vi "CR-导丝纤维毛发检测1.vi"(8 "error in (no error)":errorcluster caption="错误输入（无错误）", 11 "名称或相对路径":string="Template Program") -> (0 "error in (no error) 2":errorcluster caption="错误输入（无错误）")   [LabVIEW 2017]
uses:
  Picture/SaveButtom.ctl
  <vilib>/userdefined/High Color/IMAQdx.ctl
  <vilib>/vision/Pattern Matching.llb/IMAQ Curve Parameters.ctl
  Global System.vi
  <vilib>/Utility/xml.llb/Write to XML File(string).vi
panel:
  in  "相机选择":T1="cam0" caption="Session Out CCD3"
  in  "获取图像":bool
  in  "创建模板":bool
  in  "保存图像":bool
  out "添加的路径":path
  in  "刷新":bool
  in  "测试按钮":bool
  in  "保存按钮":bool
  in  "Main":enum32{"主参数", "颜色模板匹配参数 ", "测试效果"}(tab)
  in  "纤维毛发检测1基础参数":T2={"IsNorImage"=TRUE, "Exposure Values"=100289, "ImagePath"=path "C:/Users/hedongpo/Desktop/514-hdp/Alignment Assemble System/Test Picture/B/3.bmp", "相机选择"="cam0"} caption="参数界面" {"Exposure Values" scale=0.0..200000.0}
  in  "纤维毛发检测1参数":T4={"Curve Extraction Settings "={"Extraction Mode"=0, "Edge Threshold"=25, "Edge Filter Size"=1, "Min Length"=19, "Row Search Step Size"=5, "Col Search Step Size"=5, "Max Endpoint Gap"=10, "Closed"=FALSE, "Subpixel"=FALSE}, "Color Mode (Histogram 1)"=0, "Range (Threshold 1)"={"Lower value"=62.0, "Upper value"=255.0}, "Clamp Settings (Max Clamp 1)"={"Angle Range (+/-)"=10.0, "Edge Polarity"={"Start"=0, "End"=0}}, "Settings (Clamp (Rake) 1)"={"Contrast"=14, "Filter width"=14, "Steepness"=1, "Subsampling Ratio"=5, "Show Search Area"=FALSE, "Show Search Lines"=FALSE, "Show Edges Found"=TRUE, "Show Result"=TRUE}, "直径设定"={"Lower value"=62.0, "Upper value"=255.0}} {"Clamp Settings (Max Clamp 1)"."Edge Polarity"."Start" items=["Any", "Rising", "Falling"]; "Clamp Settings (Max Clamp 1)"."Edge Polarity"."End" items=["Any", "Rising", "Falling"]; "Color Mode (Histogram 1)" items=["RGB", "HSL", "HSV", "HSI"]; "Curve Extraction Settings"."Extraction Mode" items=["Normal", "Uniform Regions"]; "Curve Extraction Settings"."Edge Filter Size" items=["Fine", "Normal", "Contour Tracing"]; "Curve Extraction Settings"."Max Endpoint Gap" min=0; "Curve Extraction Settings"."Col Search Step Size" min=1 max=255 step=1; "Curve Extraction Settings"."Row Search Step Size" min=1 max=255 step=1; "Curve Extraction Settings"."Min Length" min=0; "Curve Extraction Settings"."Edge Threshold" min=1 max=350 step=1}
  out "结果":bool
  out "原始图像":T5(plugin-control)
  out "Distance (Clamp (Rake) 1)":sgl format="%.2f"
  out "路径输出":path
  in  "Vision Paramter Save Buttom":T6
  out "system time":string
  in  "取消按钮":bool
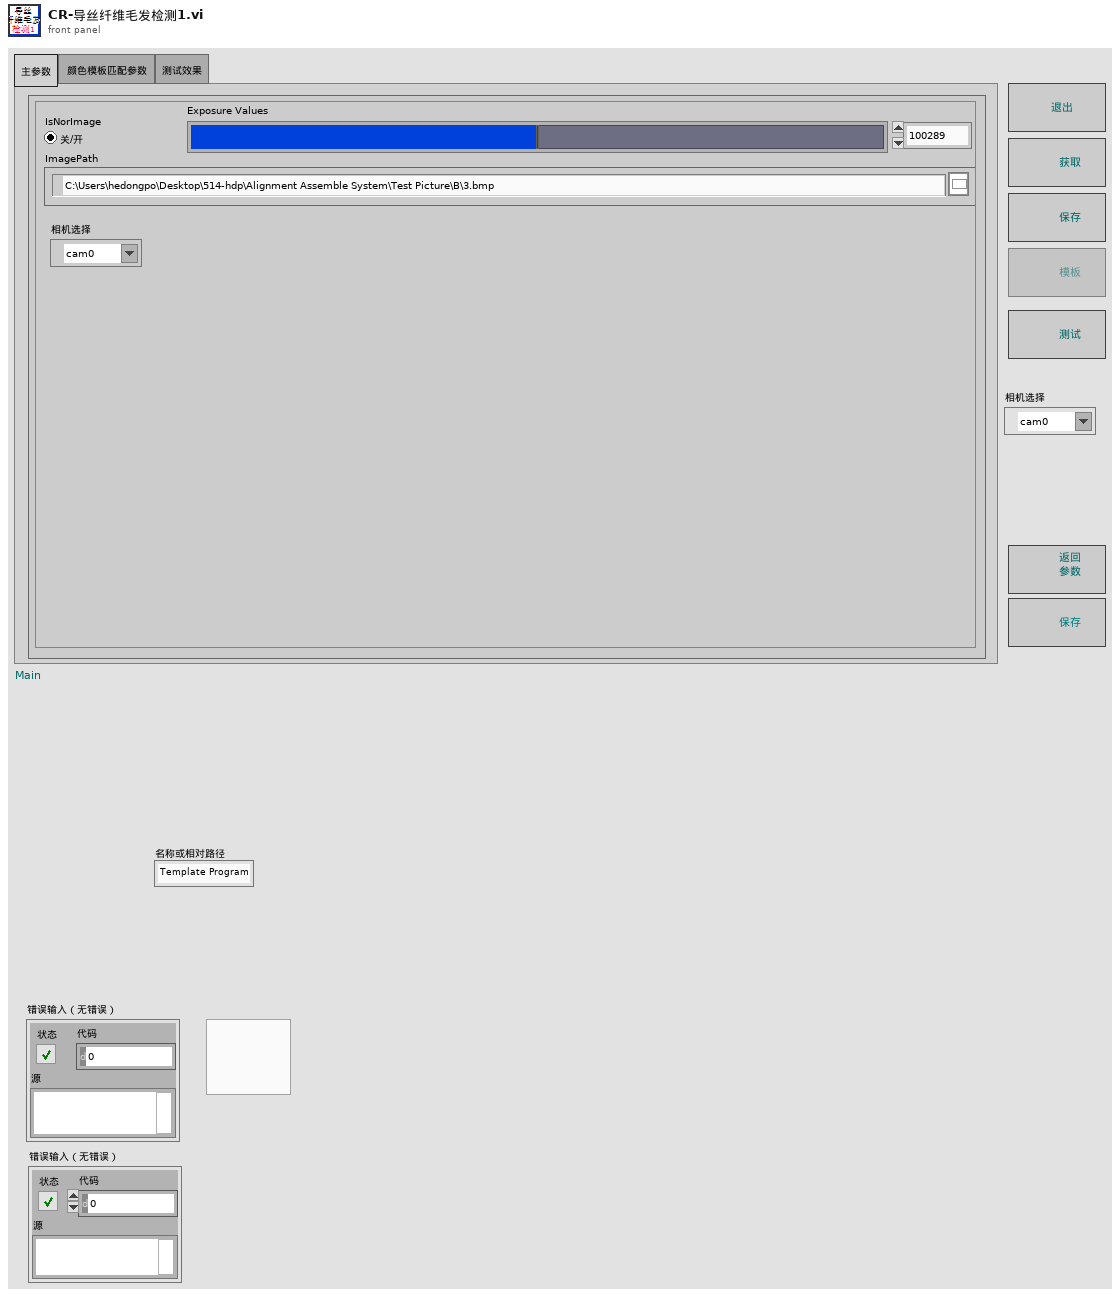
[diagram p1: front panel]
types:
  T1 = typedef "IMAQdx.ctl" = refnum<k21>
  T2 = cluster{"IsNorImage":bool, "Exposure Values":u32, "ImagePath":path, "相机选择":T1}
  T3 = typedef "IMAQ Curve Parameters.ctl" = cluster{"Extraction Mode":u32, "Edge Threshold":i32, "Edge Filter Size":u32, "Min Length":i32, "Row Search Step Size":i32, "Col Search Step Size":i32, "Max Endpoint Gap":i32, "Closed":bool, "Subpixel":bool}
  T4 = cluster{"Curve Extraction Settings ":T3, "Color Mode (Histogram 1)":u16, "Range (Threshold 1)":cluster{"Lower value":sgl, "Upper value":sgl}, "Clamp Settings (Max Clamp 1)":cluster{"Angle Range (+/-)":dbl, "Edge Polarity":cluster{"Start":u32, "End":u32}}, "Settings (Clamp (Rake) 1)":cluster{"Contrast":i32, "Filter width":i32, "Steepness":i32, "Subsampling Ratio":u32, "Show Search Area":bool, "Show Search Lines":bool, "Show Edges Found":bool, "Show Result":bool}, "直径设定":cluster{"Lower value":sgl, "Upper value":sgl}}
  T5 = typedef "IMAQ Image.ctl" = refnum<image>
  T6 = typedef "SaveButtom.ctl" = bool
  T7 = cluster{"index":i32, "this vi":refnum<vi>, "error out":errorcluster}
  T8 = cluster{"master data":string, "priority":u16, "secondary data":string[]}
  T9 = cluster{"case name":string[], "queue array":refnum<queue>[]}
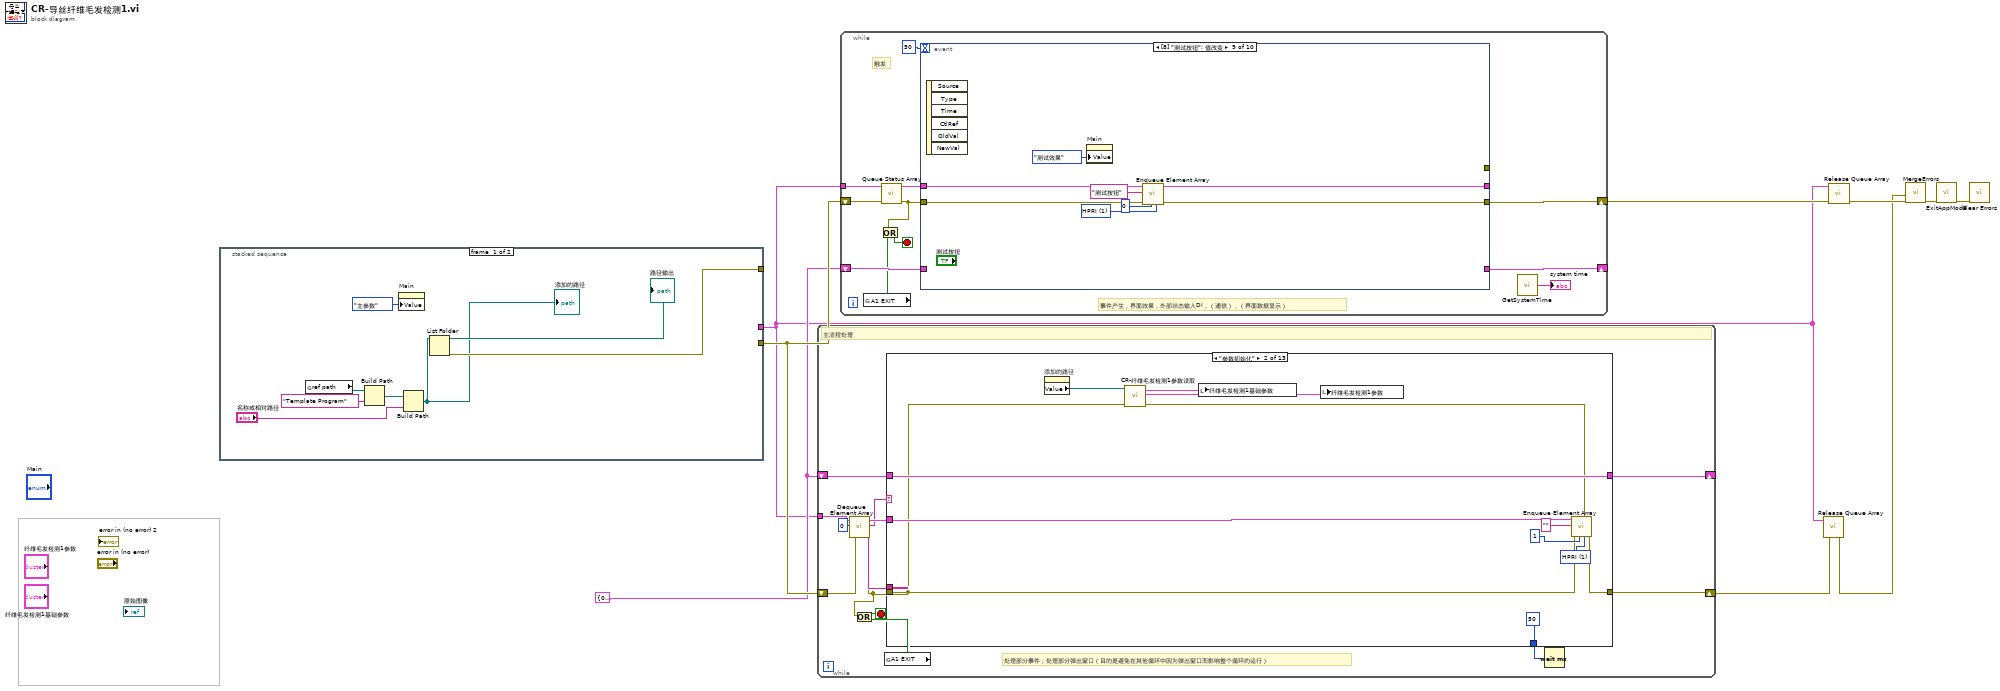
[diagram p0: block diagram]
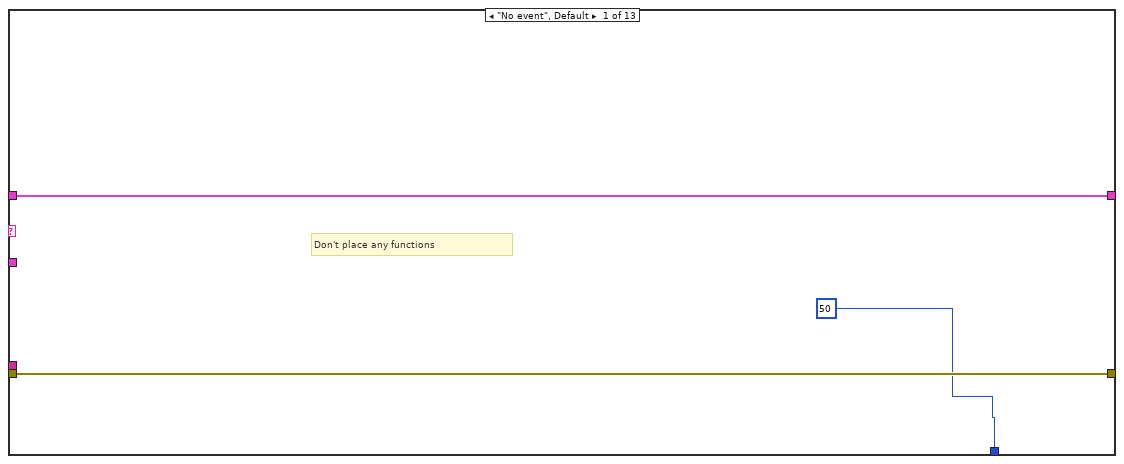
[diagram p2: hidden frame]
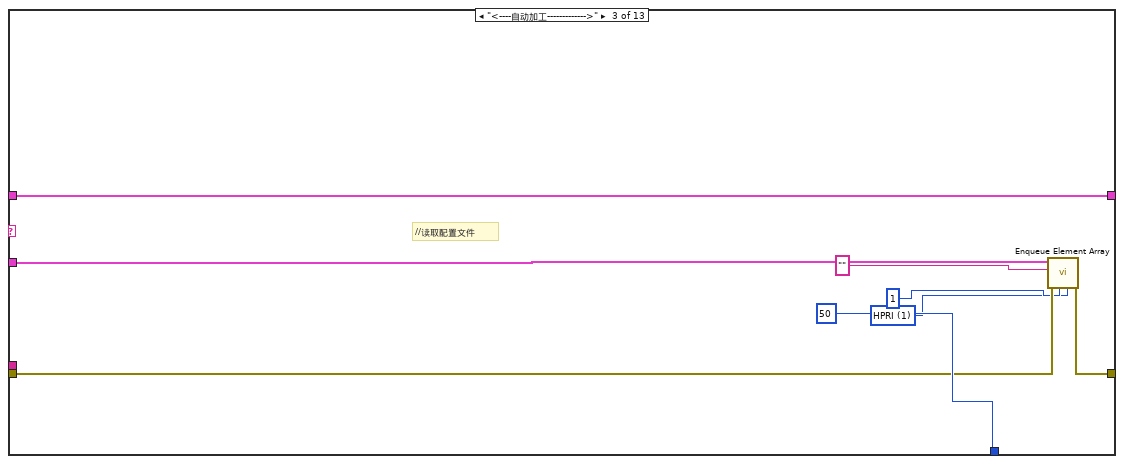
[diagram p3: hidden frame]
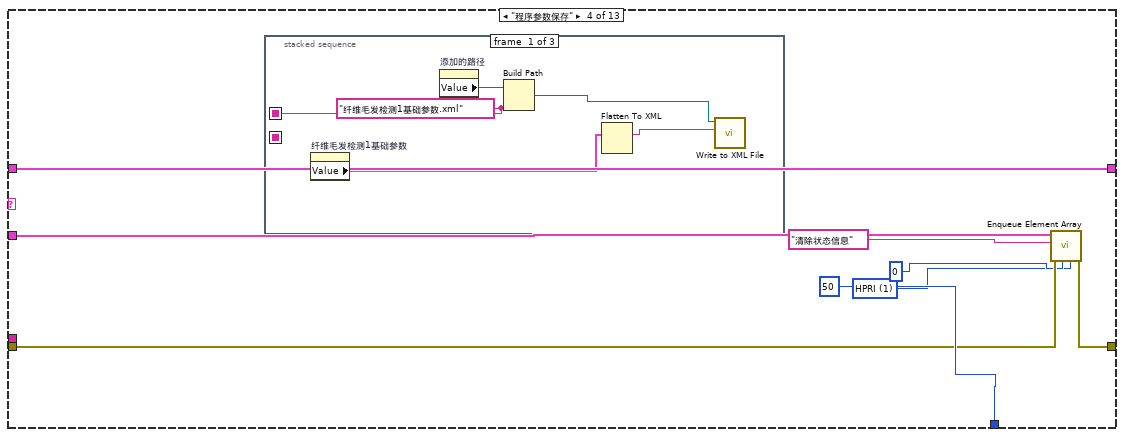
[diagram p4: hidden frame]
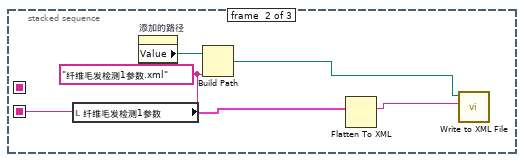
[diagram p5: hidden frame]
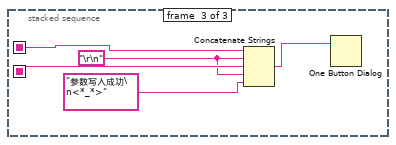
[diagram p6: hidden frame]
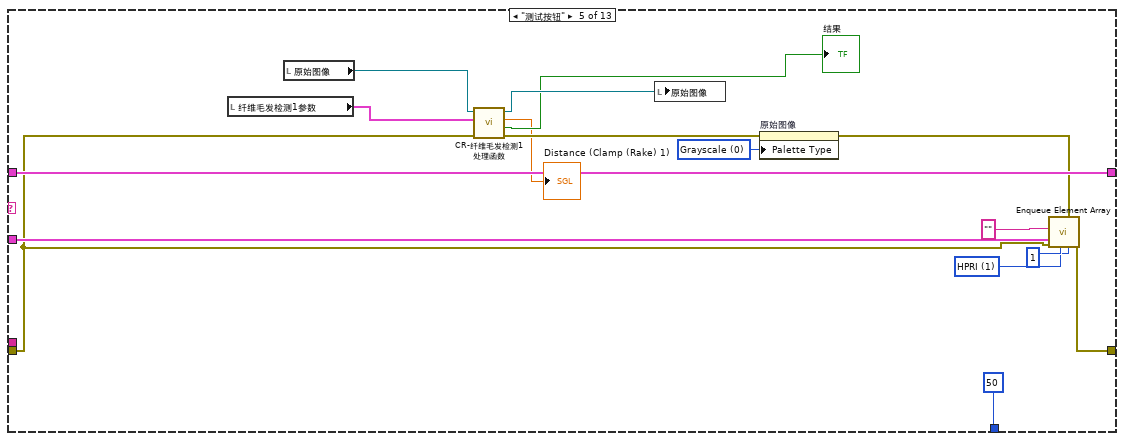
[diagram p7: hidden frame]
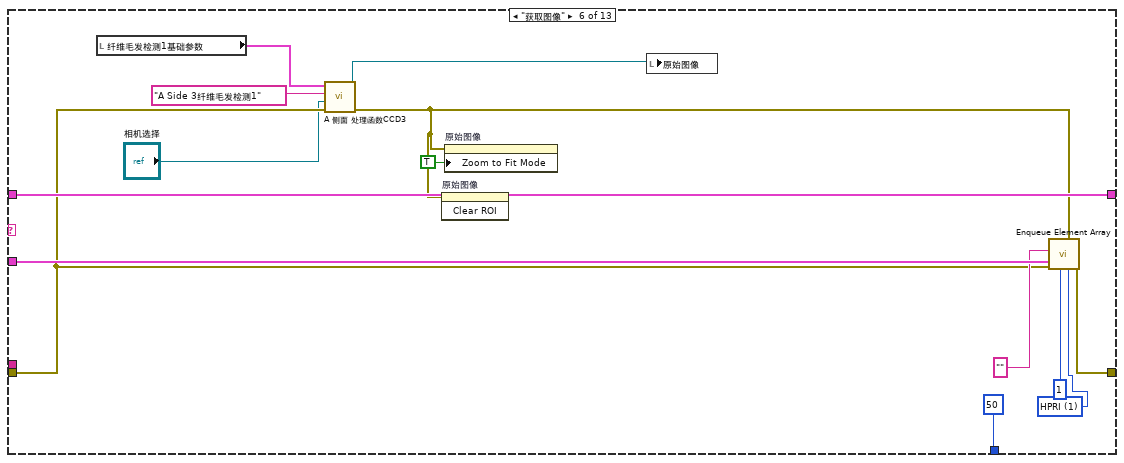
[diagram p8: hidden frame]
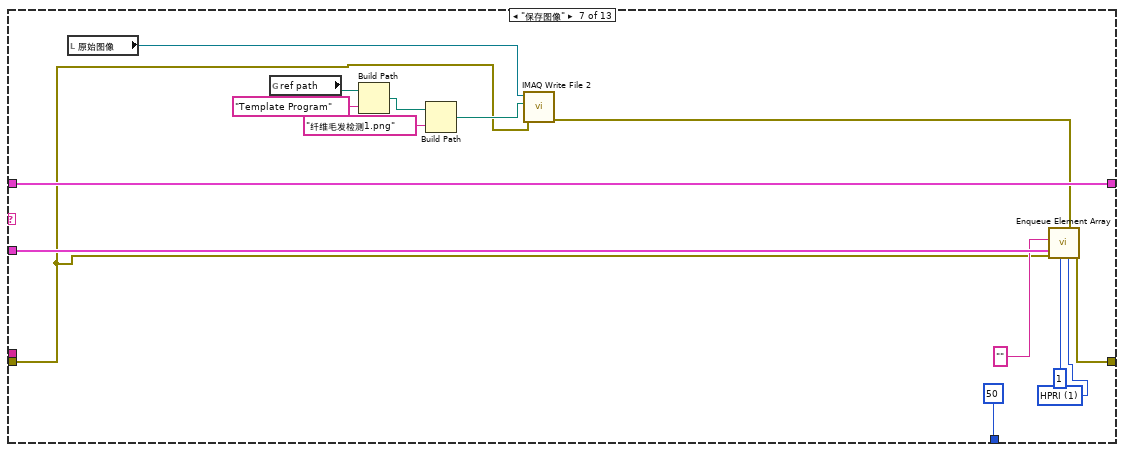
[diagram p9: hidden frame]
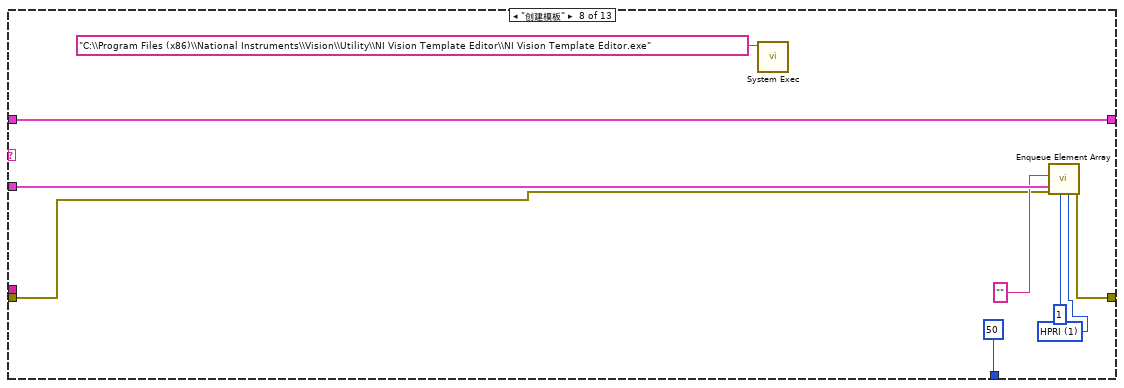
[diagram p10: hidden frame]
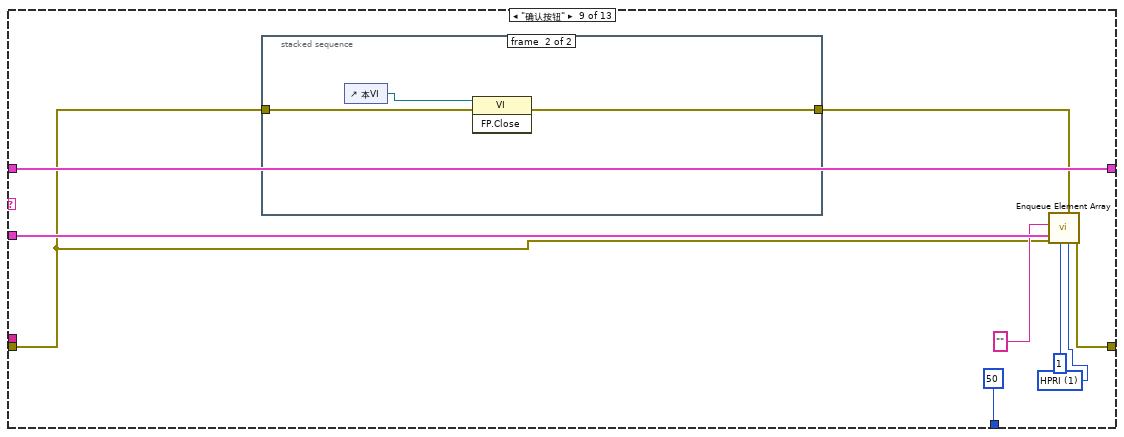
[diagram p11: hidden frame]
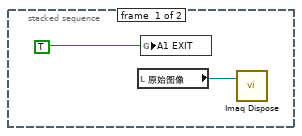
[diagram p12: hidden frame]
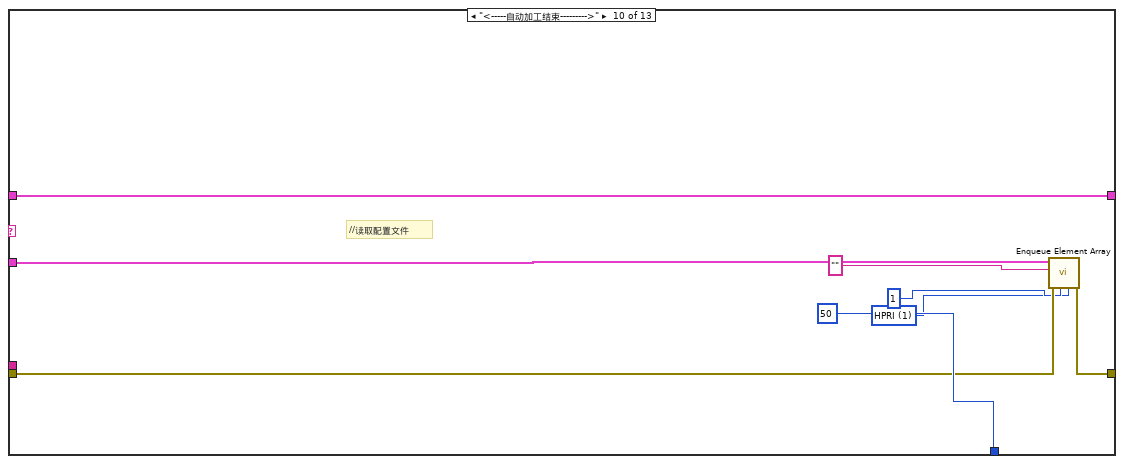
[diagram p13: hidden frame]
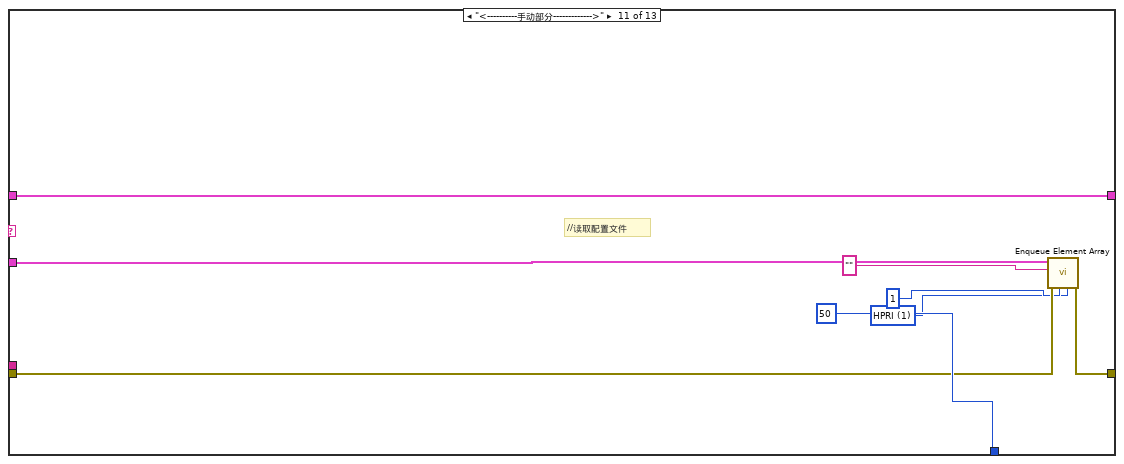
[diagram p14: hidden frame]
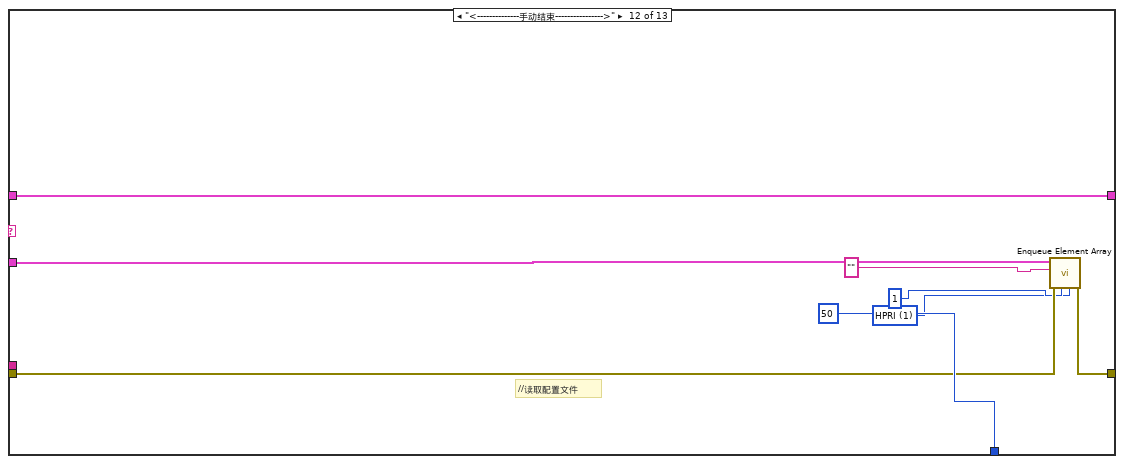
[diagram p15: hidden frame]
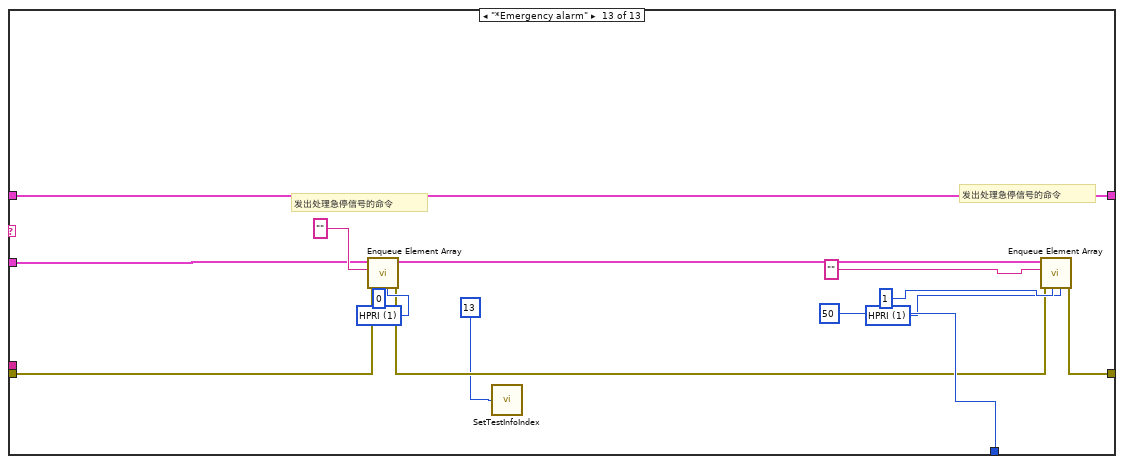
[diagram p16: hidden frame]
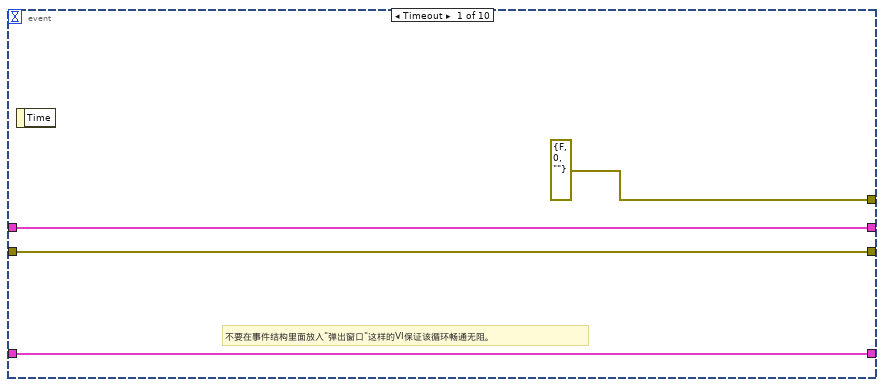
[diagram p17: hidden frame]
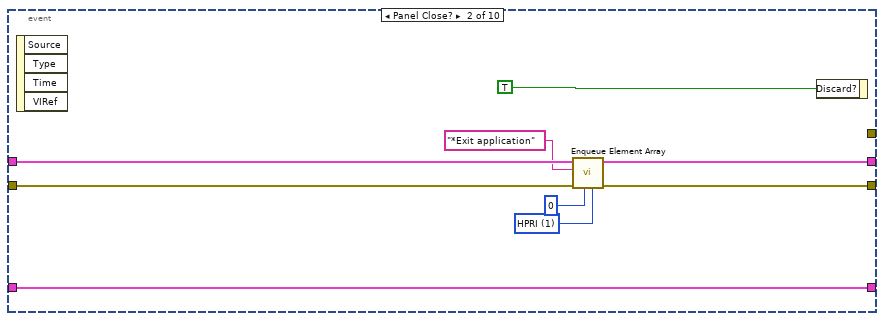
[diagram p18: hidden frame]
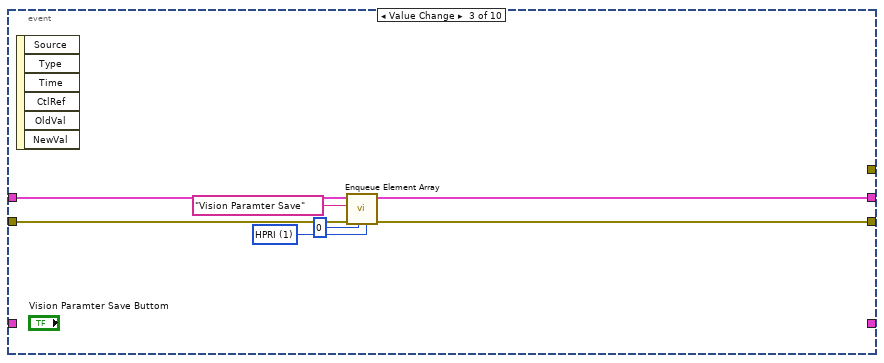
[diagram p19: hidden frame]
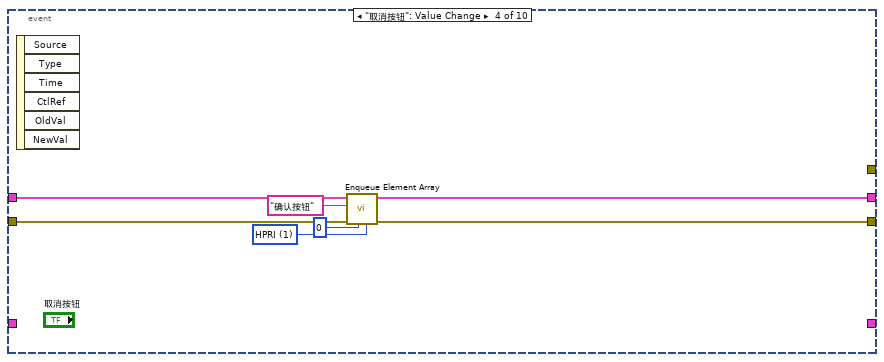
[diagram p20: hidden frame]
diagram:
  w4 = T7 {"index"=0, "this vi"=refnum, "error out"={"status"=FALSE, "code"=0, "source"=""}} ("parameter buffer")
  n1 = stacked-sequence {
    tunnel: [w16 _] -> _
    tunnel: [_ w19] -> w5
    tunnel: [_ w18] -> w1
    frame #0 {
      n2 = global read "Global System.vi" "ref path"() -> (w14:path)
      n3 = Build Path(base path=w14, name or relative path="Template Program" ("名称或相对路径")) -> (appended path=w12:path)
      n4 = property on="Main" class="TabCtl (严格)"("Value"=enum32{"主参数", "颜色模板匹配参数 ", "测试效果"}."主参数" ("Main")) -> ()  [unwired: 2 in, 2 out]
      n5 = Build Path(base path=w12, name or relative path="名称或相对路径") -> (appended path=w10:path)
      "添加的路径" <- w10
      n6 = List Folder(path=w10) -> (path out=→"路径输出":path, error out=w16:errorcluster)  [unwired: 3 in, 2 out]
    }
    frame #1 {
      w27 = string[] ["comm queue1", "data queue 11", "data queue 12", "data queue 13", "data queue 14"]  # queue name
      w28 = 4  # queue num
      w29 = T8 {"master data"="", "priority"=0, "secondary data"=[]}  # element data type
      n7 = call "Obtain Queue Array.vi"("queue name"=w27, "element data type"=w29, "queue num"=w28) -> ("error out"=w23:errorcluster, "queue out"=w24:T9)  [unwired: 2 in, 1 out]
      n8 = call "Enqueue Element Array.vi"("queue index"=0, "error in"=w23, "master data"="参数初始化", "queue in"=w24) -> ("error out"=w22:errorcluster, "queue out"=w21:T9)  [unwired: 6 in]
      n9 = disable-structure shown="启用" {
        disable-tunnel: w22 -> [w35 w36]
        disable-tunnel: w21 -> [w34 w37]
        disable-tunnel: "Loading Variable" ("master data") -> [w33 _]
        disable-tunnel: [w31 w36] -> w19
        disable-tunnel: [w30 w37] -> w18
        frame Disabled {
          n10 = call "Enqueue Element Array.vi"("queue index"=12, "error in"=w35, "master data"=w33, "queue in"=w34) -> ("error out"=w31:errorcluster, "queue out"=w30:T9)  [unwired: 6 in]
        }
        frame Enabled {
        }
      }
    }
  }
  n11 = while {
    shift-right: [w50] -> w3
    shift-left: w5 -> [w41]
    shift-right: [w47] -> _
    shift-left: w4 -> [w48]
    tunnel: w1 -> [w43]
    stop <- w38 stop-if-true
    # "处理部分事件；处理部分弹出窗口（目的是避免在其他循环中因为弹出窗口而影响整个循环的运行）"
    # "主流程处理"
    n12 = call "Dequeue Element Array.vi"("queue in"=w43, "queue index"=0, "error in"=w41) -> ("queue out"=w46:T9, "master data"=w45:string, "secondary data"=w44:string[], "error out"=w40:errorcluster)  [unwired: 2 in, 1 out]
    n13 = global read "Global System.vi" "A1 EXIT"() -> (w39:bool)
    n14 = Or(x=w40, y=w39) -> (x .or. y?=w38:bool)
    n15 = case shown="\"参数初始化\"" w45 {
      tunnel: w46 -> [_ w64 w72 w74 w111 w125 w140 w149 w158 w171 w179 w187 w193]
      tunnel: w40 -> [w52 w58 w68 w78 w103 w116 w127 w143 w152 w167 w175 w183 w190]
      tunnel: [w52 w63 w71 w80 w110 w124 w139 w148 w157 w170 w178 w186 w201] -> w50
      tunnel: [50 50 50 50 50 50 50 50 50 50 50 50 50] -> w49
      tunnel: w48 -> [w53 w59 w69 w75 w106 w120 w135 w144 w153 w168 w176 w184 w199]
      tunnel: [w53 w59 w69 w75 w106 w120 w135 w144 w153 w168 w176 w184 w199] -> w47
      tunnel: w44 -> [_ _ _ _ _ _ _ _ _ _ _ _ _]
      frame "No event", Default {
        # "Don't place any functions"
      }
      frame "参数初始化" {
        w60 = u16 1 items=["HPRI"=1, "LPRI"=0] ("priority")
        n16 = property on="添加的路径" class="Path"() -> ("Value"=w56:path)  [unwired: 2 in, 2 out]
        n17 = call "CR-纤维毛发检测1参数读取.vi"("error in (no error)"=w58, "基路径"=w56) -> ("error out"=w57:errorcluster, "纤维毛发检测1参数"=w54:T4, "纤维毛发检测1基础参数"=w55:T2)  [unwired: 6 in]
        n18 = local write "纤维毛发检测1基础参数"(w55) -> ()
        n19 = local write "纤维毛发检测1参数"(w54) -> ()
        n20 = call "Enqueue Element Array.vi"("priority"=w60, "device error in"=w57, "queue index"=1, "error in"=w58, "master data"="" ("Element 1"), "queue in"=w64) -> ("error out"=w63:errorcluster)  [unwired: 4 in, 1 out]
      }
      frame "<----自动加工------------->" {
        w66 = u16 1 items=["HPRI"=1, "LPRI"=0] ("priority")
        # "//读取配置文件"
        n21 = call "Enqueue Element Array.vi"("priority"=w66, "queue index"=1, "error in"=w68, "master data"="" ("Element 1"), "queue in"=w72) -> ("error out"=w71:errorcluster)  [unwired: 5 in, 1 out]
      }
      frame "程序参数保存" {
        w76 = u16 1 items=["HPRI"=1, "LPRI"=0] ("priority")
        n22 = stacked-sequence {
          seq-local: [w82 _ _] -> [_ _ w95]
          seq-local: [_ w88 _] -> [_ _ w93]
          frame #0 {
            w82 = "纤维毛发检测1基础参数.xml" ("名称或相对路径")
            n23 = property on="纤维毛发检测1基础参数" class="Clust (严格)"() -> ("Value"=w85:T2)  [unwired: 2 in, 2 out]
            n24 = property on="添加的路径" class="Path"() -> ("Value"=w86:path)  [unwired: 2 in, 2 out]
            n25 = Build Path(base path=w86, name or relative path=w82) -> (appended path=w83:path)
            n26 = Flatten To XML(anything=w85) -> (xml string=w84:string)
            n27 = call-poly <vilib>:"Write to XML File.vi"("XML Input"=w84, "XML File Path"=w83) -> ()  [unwired: 7 in, 3 out]
          }
          frame #1 {
            w88 = "纤维毛发检测1参数.xml" ("名称或相对路径")
            n28 = local read "纤维毛发检测1参数"() -> (w87:T4)
            n29 = property on="添加的路径" class="Path"() -> ("Value"=w91:path)  [unwired: 2 in, 2 out]
            n30 = Build Path(base path=w91, name or relative path=w88) -> (appended path=w89:path)
            n31 = Flatten To XML(anything=w87) -> (xml string=w90:string)
            n32 = call-poly <vilib>:"Write to XML File.vi"("XML Input"=w90, "XML File Path"=w89) -> ()  [unwired: 7 in, 3 out]
          }
          frame #2 {
            w92 = "\r\n"
            n33 = Concatenate Strings(w95, w92, w93, w92, "参数写入成功\n<*_*>" ("消息")) -> (w94:string)
            n34 = One Button Dialog(message=w94) -> ()  [unwired: 1 in, 1 out]
          }
        }
        n35 = call "Enqueue Element Array.vi"("priority"=w76, "queue index"=0, "error in"=w78, "master data"="清除状态信息" ("Element 1"), "queue in"=w74) -> ("error out"=w80:errorcluster)  [unwired: 5 in, 1 out]
      }
      frame "测试按钮" {
        w100 = u32 0 items=["Grayscale", "Binary", "Gradient", "Rainbow", "Temperature", "User Defined", "Binary 16 Bit", "Gradient 16 Bit", "Rainbow 16 Bit", "Temperature 16 Bit", "User Defined 16 Bit"] ("Palette:Palette Type")
        w107 = u16 1 items=["HPRI"=1, "LPRI"=0] ("priority")
        n36 = local read "纤维毛发检测1参数"() -> (w99:T4)
        n37 = local read "原始图像"() -> (w105:T5)
        n38 = call "CR-纤维毛发检测1处理函数.vi"("error in (no error)"=w103, "UI电源线正面漏线参数"=w99, "Image in"=w105) -> ("error out"=w102:errorcluster, "纤维毛发"=→"结果":bool, "Distance (Clamp (Rake) 1)"=→"Distance (Clamp (Rake) 1)":sgl, "Image out"=w104:T5)  [unwired: 4 in, 1 out]
        n39 = local write "原始图像"(w104) -> ()
        n40 = property on="原始图像" class="ImageControl"(error in=w102, "Palette Type"=w100) -> (error out=w101:errorcluster)  [unwired: 1 in, 1 out]
        n41 = call "Enqueue Element Array.vi"("priority"=w107, "device error in"=w101, "queue index"=1, "error in"=w103, "master data"="" ("Element 1"), "queue in"=w111) -> ("error out"=w110:errorcluster)  [unwired: 4 in, 1 out]
      }
      frame "获取图像" {
        w121 = u16 1 items=["HPRI"=1, "LPRI"=0] ("priority")
        n42 = local read "纤维毛发检测1基础参数"() -> (w118:T2)
        n43 = call "A 侧面 处理函数CCD3.vi"("error in (no error)"=w116, "相机选择"="相机选择", "New Image"="A Side 3纤维毛发检测1" ("Image Name"), "ParamsUI"=w118) -> ("error out"=w114:errorcluster, "Image out"=w117:T5)  [unwired: 4 in, 2 out]
        n44 = invoke on="原始图像" class="ImageControl" method="Clear ROI"(error in=w114) -> ()  [unwired: 2 in, 3 out]
        n45 = property on="原始图像" class="ImageControl"(error in=w114, "Zoom to Fit Mode"=TRUE) -> ()  [unwired: 1 in, 2 out]
        n46 = local write "原始图像"(w117) -> ()
        n47 = call "Enqueue Element Array.vi"("priority"=w121, "device error in"=w114, "queue index"=1, "error in"=w116, "master data"="" ("Element 1"), "queue in"=w125) -> ("error out"=w124:errorcluster)  [unwired: 4 in, 1 out]
      }
      frame "保存图像" {
        w136 = u16 1 items=["HPRI"=1, "LPRI"=0] ("priority")
        n48 = local read "原始图像"() -> (w128:T5)
        n49 = global read "Global System.vi" "ref path"() -> (w134:path)
        n50 = Build Path(base path=w134, name or relative path="Template Program" ("名称或相对路径")) -> (appended path=w132:path)
        n51 = Build Path(base path=w132, name or relative path="纤维毛发检测1.png" ("名称或相对路径")) -> (appended path=w130:path)
        n52 = call-poly "IMAQ Write File 2"("error in (no error)"=w127, "File Path"=w130, "Image"=w128) -> ("error out"=w129:errorcluster)  [unwired: 7 in, 1 out]
        n53 = call "Enqueue Element Array.vi"("priority"=w136, "device error in"=w129, "queue index"=1, "error in"=w127, "master data"="" ("Element 1"), "queue in"=w140) -> ("error out"=w139:errorcluster)  [unwired: 4 in, 1 out]
      }
      frame "创建模板" {
        w145 = u16 1 items=["HPRI"=1, "LPRI"=0] ("priority")
        n54 = call <vilib>:"System Exec.vi"("command line"="C:\\Program Files (x86)\\National Instruments\\Vision\\Utility\\NI Vision Template Editor\\NI Vision Template Editor.exe") -> ()  [unwired: 7 in, 4 out]
        n55 = call "Enqueue Element Array.vi"("priority"=w145, "queue index"=1, "error in"=w143, "master data"="" ("Element 1"), "queue in"=w149) -> ("error out"=w148:errorcluster)  [unwired: 5 in, 1 out]
      }
      frame "确认按钮" {
        w154 = u16 1 items=["HPRI"=1, "LPRI"=0] ("priority")
        n56 = stacked-sequence {
          tunnel: w152 -> [_ w163]
          tunnel: [_ w162] -> w151
          frame #0 {
            n57 = local read "原始图像"() -> (w160:T5)
            n58 = global write "Global System.vi" "A1 EXIT"(TRUE ("EXIT")) -> ()
            n59 = call "Imaq Dispose"("Image"=w160) -> ()  [unwired: 5 in, 1 out]
          }
          frame #1 {
            n60 = control-ref of="本VI"() -> (w164:refnum<vi>)
            n61 = invoke class="VI" method="FP.Close"(reference=w164, error in=w163) -> (error out=w162:errorcluster)  [unwired: 1 in, 2 out]
          }
        }
        n62 = call "Enqueue Element Array.vi"("priority"=w154, "device error in"=w151, "queue index"=1, "error in"=w152, "master data"="" ("Element 1"), "queue in"=w158) -> ("error out"=w157:errorcluster)  [unwired: 4 in, 1 out]
      }
      frame "<-----自动加工结束--------->" {
        w165 = u16 1 items=["HPRI"=1, "LPRI"=0] ("priority")
        # "//读取配置文件"
        n63 = call "Enqueue Element Array.vi"("priority"=w165, "queue index"=1, "error in"=w167, "master data"="" ("Element 1"), "queue in"=w171) -> ("error out"=w170:errorcluster)  [unwired: 5 in, 1 out]
      }
      frame "<----------手动部分------------->" {
        w173 = u16 1 items=["HPRI"=1, "LPRI"=0] ("priority")
        # "//读取配置文件"
        n64 = call "Enqueue Element Array.vi"("priority"=w173, "queue index"=1, "error in"=w175, "master data"="" ("Element 1"), "queue in"=w179) -> ("error out"=w178:errorcluster)  [unwired: 5 in, 1 out]
      }
      frame "<--------------手动结束---------------->" {
        w181 = u16 1 items=["HPRI"=1, "LPRI"=0] ("priority")
        # "//读取配置文件"
        n65 = call "Enqueue Element Array.vi"("priority"=w181, "queue index"=1, "error in"=w183, "master data"="" ("Element 1"), "queue in"=w187) -> ("error out"=w186:errorcluster)  [unwired: 5 in, 1 out]
      }
      frame "*Emergency alarm" {
        w196 = u16 1 items=["HPRI"=1, "LPRI"=0] ("priority")
        w197 = u16 1 items=["HPRI"=1, "LPRI"=0] ("priority")
        # "发出处理急停信号的命令"
        # "发出处理急停信号的命令"
        n66 = call "Enqueue Element Array.vi"("priority"=w196, "queue index"=0, "error in"=w190, "master data"="" ("Element 1"), "queue in"=w193) -> ("error out"=w191:errorcluster, "queue out"=w192:T9)  [unwired: 5 in]
        n67 = call "SetTestInfoIndex.vi"("test info index"=13) -> ()
        n68 = call "Enqueue Element Array.vi"("priority"=w197, "queue index"=1, "error in"=w191, "master data"="" ("Element 1"), "queue in"=w192) -> ("error out"=w201:errorcluster)  [unwired: 5 in, 1 out]
      }
    }
    n69 = Wait (ms)(milliseconds to wait=w49) -> ()  [unwired: 1 out]
  }
  n70 = while {
    shift-right: [w206] -> w6
    shift-left: w5 -> [w210]
    shift-right: [w208] -> _
    shift-left: w4 -> [w209]
    tunnel: w1 -> [w212]
    stop <- w203 stop-if-true
    # "触发"
    # "事件产生，界面效果，外部状态输入DI，（通信），（界面数据显示）"
    n71 = global read "Global System.vi" "A1 EXIT"() -> (w204:bool)
    n72 = call "Queue Status Array.vi"("error in (no error)"=w210, "queue in"=w212) -> ("error out"=w205:errorcluster, "queue out"=w207:T9)  [unwired: 4 in]
    n73 = Or(x=w205, y=w204) -> (x .or. y?=w203:bool)
    n74 = event shown="[8] \"测试按钮\": 值改变" {
      selector: _ -> [_ _ _ _ _ _ _ _ _ _]
      dyn-events: _ -> [_ _ _ _ _ _ _ _ _ _]
      timeout: 50 -> [_ _ _ _ _ _ _ _ _ _]
      tunnel: w209 -> [w217 w225 _ _ _ _ _ _ _ _]
      tunnel: [w217 w225 _ _ _ _ _ _ _ _] -> w208
      tunnel: [errorcluster {"status"=FALSE, "code"=0, "source"=""} ("error out") _ _ _ _ _ _ _ _ _] -> _
      tunnel: w207 -> [w215 w224 w230 w237 w244 w252 w259 w266 w274 w282]
      tunnel: w205 -> [w214 w223 w229 w236 w243 w251 w258 w265 w273 w281]
      tunnel: [w214 w222 w227 w234 w241 w249 w256 w263 w271 w279] -> w206
      tunnel: [w215 w221 w228 w235 w242 w250 w257 w264 w272 w280] -> _
      event Timeout {
        # "不要在事件结构里面放入\"弹出窗口\"这样的VI保证该循环畅通无阻。"
        n75 = event-data() -> ()  [unwired: 1 in, 1 out]
      }
      event Panel Close? {
        w219 = u16 1 items=["HPRI"=1, "LPRI"=0] ("priority")
        n76 = event-data() -> ()  [unwired: 1 in, 4 out]
        n77 = call "Enqueue Element Array.vi"("priority"=w219, "queue index"=0, "error in"=w223, "master data"="*Exit application", "queue in"=w224) -> ("error out"=w222:errorcluster, "queue out"=w221:T9)  [unwired: 5 in]
        n78 = event-data("Discard?"=TRUE) -> ()  [unwired: 1 in, 1 out]
      }
      event Value Change {
        w232 = u16 1 items=["HPRI"=1, "LPRI"=0] ("priority")
        n79 = event-data() -> ()  [unwired: 1 in, 6 out]
        n80 = call "Enqueue Element Array.vi"("priority"=w232, "queue index"=0, "error in"=w229, "master data"="Vision Paramter Save", "queue in"=w230) -> ("error out"=w227:errorcluster, "queue out"=w228:T9)  [unwired: 5 in]
      }
      event "取消按钮": Value Change {
        w239 = u16 1 items=["HPRI"=1, "LPRI"=0] ("priority")
        n81 = event-data() -> ()  [unwired: 1 in, 6 out]
        n82 = call "Enqueue Element Array.vi"("priority"=w239, "queue index"=0, "error in"=w236, "master data"="确认按钮", "queue in"=w237) -> ("error out"=w234:errorcluster, "queue out"=w235:T9)  [unwired: 5 in]
      }
      event "保存按钮": Value Change {
        w246 = u16 1 items=["HPRI"=1, "LPRI"=0] ("priority")
        n83 = event-data() -> ()  [unwired: 1 in, 6 out]
        n84 = call "Enqueue Element Array.vi"("priority"=w246, "queue index"=0, "error in"=w243, "master data"="程序参数保存", "queue in"=w244) -> ("error out"=w241:errorcluster, "queue out"=w242:T9)  [unwired: 5 in]
      }
      event "获取图像": Value Change {
        w254 = u16 1 items=["HPRI"=1, "LPRI"=0] ("priority")
        n85 = event-data() -> ()  [unwired: 1 in, 6 out]
        n86 = property on="Main" class="TabCtl (严格)"("Value"=enum32{"主参数", "颜色模板匹配参数 ", "测试效果"}."测试效果" ("Main")) -> ()  [unwired: 2 in, 2 out]
        n87 = call "Enqueue Element Array.vi"("priority"=w254, "queue index"=0, "error in"=w251, "master data"="获取图像", "queue in"=w252) -> ("error out"=w249:errorcluster, "queue out"=w250:T9)  [unwired: 5 in]
      }
      event "保存图像": Value Change {
        w261 = u16 1 items=["HPRI"=1, "LPRI"=0] ("priority")
        n88 = event-data() -> ()  [unwired: 1 in, 6 out]
        n89 = call "Enqueue Element Array.vi"("priority"=w261, "queue index"=0, "error in"=w258, "master data"="保存图像", "queue in"=w259) -> ("error out"=w256:errorcluster, "queue out"=w257:T9)  [unwired: 5 in]
      }
      event "创建模板": Value Change {
        w268 = u16 1 items=["HPRI"=1, "LPRI"=0] ("priority")
        n90 = event-data() -> ()  [unwired: 1 in, 6 out]
        n91 = call "Enqueue Element Array.vi"("priority"=w268, "queue index"=0, "error in"=w265, "master data"="创建模板", "queue in"=w266) -> ("error out"=w263:errorcluster, "queue out"=w264:T9)  [unwired: 5 in]
      }
      event "测试按钮": Value Change {
        w276 = u16 1 items=["HPRI"=1, "LPRI"=0] ("priority")
        n92 = event-data() -> ()  [unwired: 1 in, 6 out]
        n93 = property on="Main" class="TabCtl (严格)"("Value"=enum32{"主参数", "颜色模板匹配参数 ", "测试效果"}."测试效果" ("Main")) -> ()  [unwired: 2 in, 2 out]
        n94 = call "Enqueue Element Array.vi"("priority"=w276, "queue index"=0, "error in"=w273, "master data"="测试按钮", "queue in"=w274) -> ("error out"=w271:errorcluster, "queue out"=w272:T9)  [unwired: 5 in]
      }
      event "刷新": Value Change {
        n95 = event-data() -> ()  [unwired: 1 in, 6 out]
        n96 = disable-structure shown="禁用" {
          disable-tunnel: w282 -> [w286 _]
          disable-tunnel: w281 -> [w285 _]
          disable-tunnel: [w284 _] -> w280
          disable-tunnel: [w283 _] -> w279
          frame Disabled {
            w288 = u16 1 items=["HPRI"=1, "LPRI"=0] ("priority")
            # "刷新"
            n97 = call "Enqueue Element Array.vi"("priority"=w288, "queue index"=0, "error in"=w285, "master data"="刷新", "queue in"=w286) -> ("error out"=w283:errorcluster, "queue out"=w284:T9)  [unwired: 5 in]
          }
          frame Enabled {
          }
        }
        n98 = property on="Main" class="TabCtl (严格)"("Value"=enum32{"主参数", "颜色模板匹配参数 ", "测试效果"}."颜色模板匹配参数 " ("Main")) -> ()  [unwired: 2 in, 2 out]
      }
    }
    n99 = call "GetSystemTime.vi"() -> ("date/time string"=→"system time":string)  [unwired: 7 in]
  }
  n100 = call "Release Queue Array.vi"("error in"=w3, "queue in"=w1) -> ("error out"=w2:errorcluster)  [unwired: 2 in, 3 out]
  n101 = call "Release Queue Array.vi"("error in"=w6, "queue in"=w1) -> ("error out"=w9:errorcluster)  [unwired: 2 in, 3 out]
  n102 = call "MergeErrors.vi"("error in 3 (no error)"=w2, "error in 4 (no error)"=w9) -> ("error out"=w8:errorcluster)  [unwired: 6 in]
  n103 = call "ExitAppMode.vi"("error in (no error)"=w8) -> ("error out"=w7:errorcluster)  [unwired: 10 in]
  n104 = call <vilib>:"Clear Errors.vi"("error in (no error)"=w7) -> ()  [unwired: 5 in, 2 out]
